vi "python简单的加法器.vi"() -> ()   [LabVIEW 2022 SP3]
panel:
  out "返回值":dbl
  out "error out":errorcluster
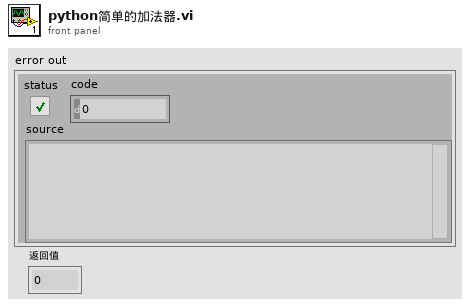
[diagram p1: front panel]
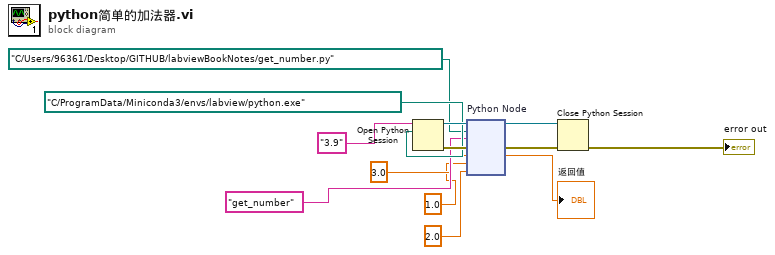
[diagram p0: block diagram]
diagram:
  n1 = Open Python Session(python version="3.9" ("Python版本"), python path=path "C:/ProgramData/Miniconda3/envs/labview/python.exe" ("Python路径")) -> (session out=w8:refnum<k35>, error out=w9:errorcluster)  [unwired: 1 in]
  n2 = node "Python Node"(w8, path "C:/Users/96361/Desktop/GITHUB/labviewBookNotes/get_number.py" ("模块路径"), "get_number" ("函数名称"), w9, 3.0, 1.0, 2.0) -> (w13:refnum<k35>, w12:errorcluster, →"返回值":dbl)  [unwired: 2 in, 2 out]
  n3 = Close Python Session(session in=w13, error in=w12) -> (11:→"error out":errorcluster)
